vi "RUSHArmControl.vi"(1 "In Cluster":T2) -> (0 "Out Cluster":T1)   [LabVIEW 2012]
panel:
  in  "Setpoint P Gain":dbl=2.0
  in  "Manual P Gain":dbl=2.0
  in  "Vision P Gain":dbl=0.75
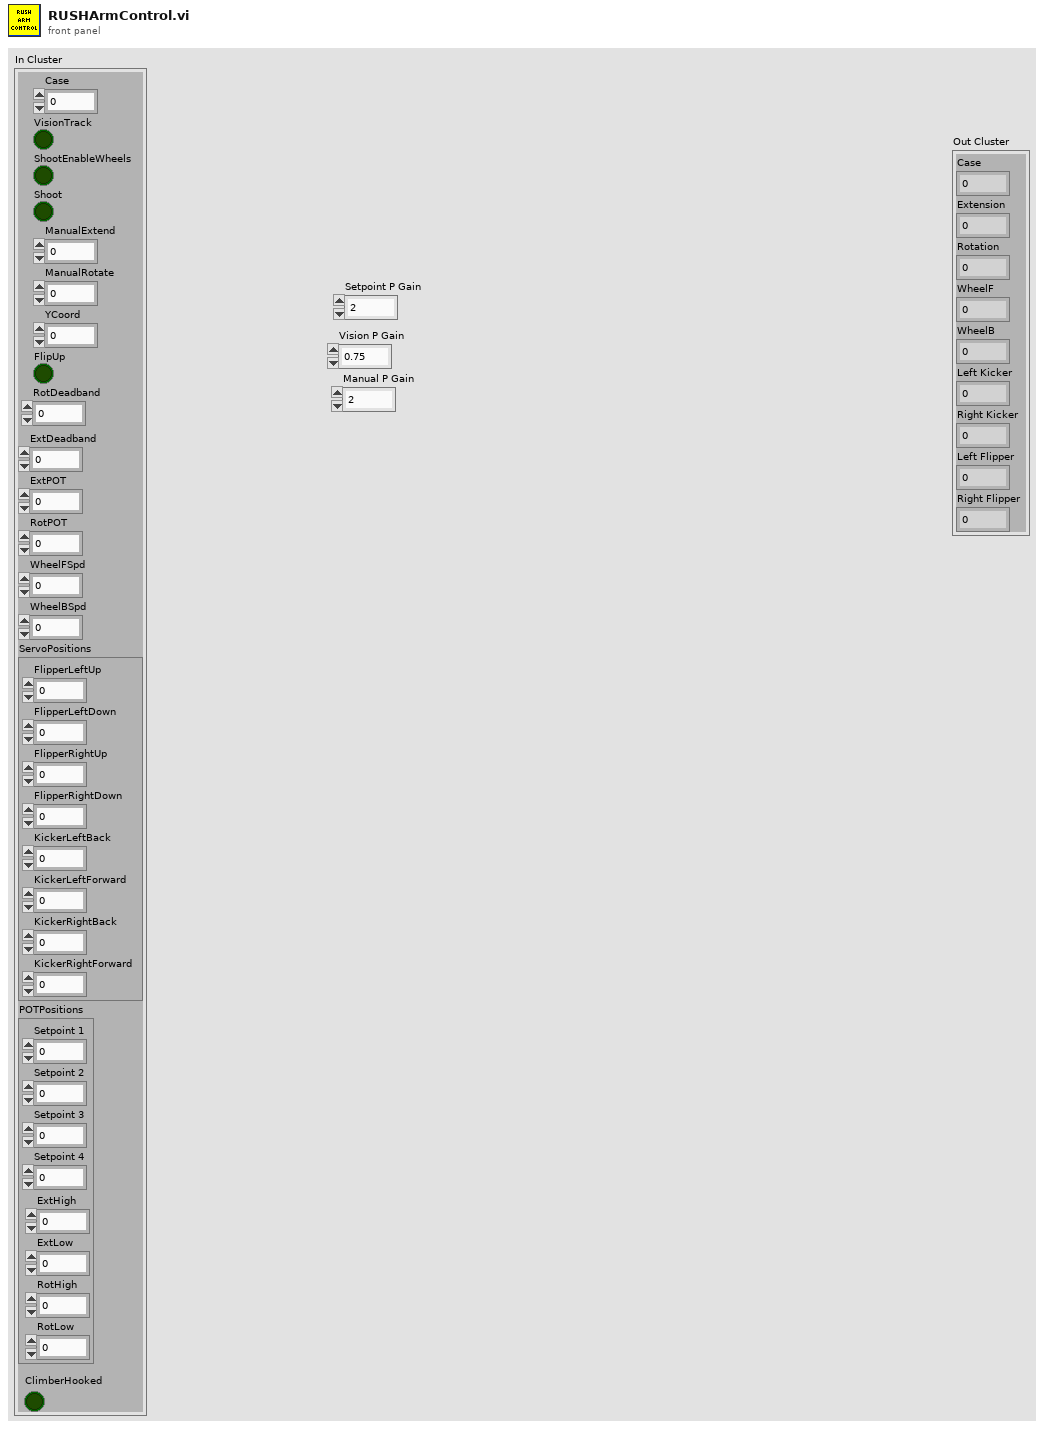
[diagram p1: front panel]
types:
  T1 = cluster{"Case":dbl, "Extension":dbl, "Rotation":dbl, "WheelF":dbl, "WheelB":dbl, "Left Kicker":dbl, "Right Kicker":dbl, "Left Flipper":dbl, "Right Flipper":dbl}
  T2 = cluster{"Case":dbl, "VisionTrack":bool, "ShootEnableWheels":bool, "Shoot":bool, "ManualExtend":dbl, "ManualRotate":dbl, "YCoord":dbl, "FlipUp":bool, "RotDeadband":dbl, "ExtDeadband":dbl, "ExtPOT":dbl, "RotPOT":dbl, "WheelFSpd":dbl, "WheelBSpd":dbl, "ServoPositions":cluster{"FlipperLeftUp":dbl, "FlipperLeftDown":dbl, "FlipperRightUp":dbl, "FlipperRightDown":dbl, "KickerLeftBack":dbl, "KickerLeftForward":dbl, "KickerRightBack":dbl, "KickerRightForward":dbl}, "POTPositions":cluster{"Setpoint 1":dbl, "Setpoint 2":dbl, "Setpoint 3":dbl, "Setpoint 4":dbl, "RotLow":dbl, "RotHigh":dbl, "ExtLow":dbl, "ExtHigh":dbl}, "ClimberHooked":bool}
  T3 = cluster{"FlipperLeftUp":dbl, "FlipperLeftDown":dbl, "FlipperRightUp":dbl, "FlipperRightDown":dbl, "KickerLeftBack":dbl, "KickerLeftForward":dbl, "KickerRightBack":dbl, "KickerRightForward":dbl}
  T4 = cluster{"Setpoint 1":dbl, "Setpoint 2":dbl, "Setpoint 3":dbl, "Setpoint 4":dbl, "RotLow":dbl, "RotHigh":dbl, "ExtLow":dbl, "ExtHigh":dbl}
  T5 = cluster{"t":dbl, "y":dbl, "y":dbl, "Output":dbl, "Output":dbl, "KickerLeftBack":dbl, "KickerRightBack":dbl, "FlipperLeftDown":dbl, "FlipperRightDown":dbl}
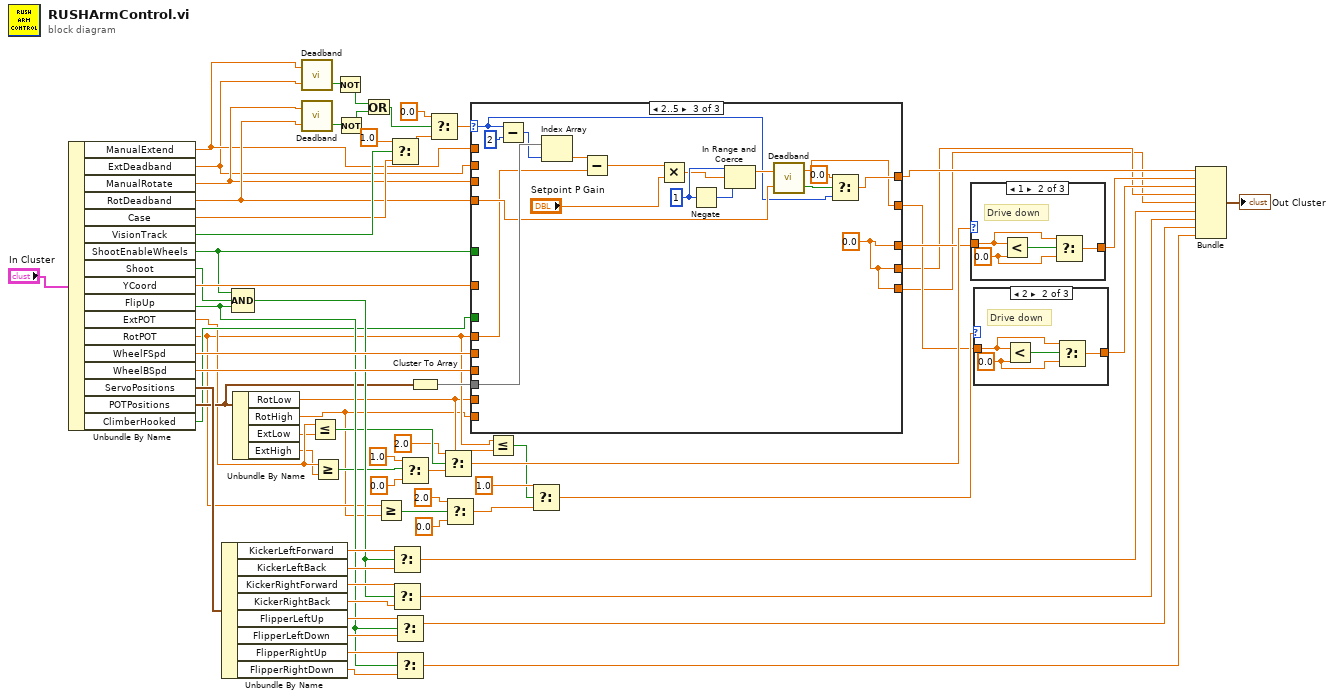
[diagram p0: block diagram]
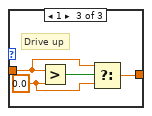
[diagram p3: hidden frame]
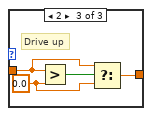
[diagram p5: hidden frame]
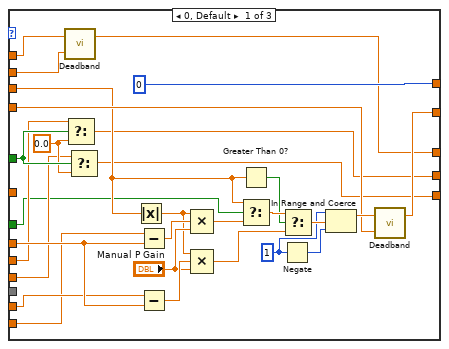
[diagram p6: hidden frame]
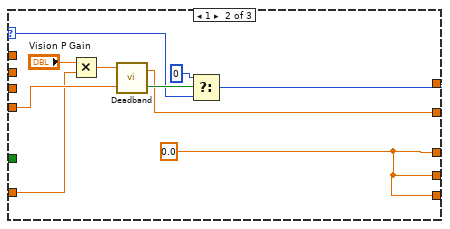
[diagram p7: hidden frame]
diagram:
  n1 = Unbundle By Name("In Cluster") -> ("ManualExtend"=w52:dbl, "ExtDeadband"=w51:dbl, "ManualRotate"=w53:dbl, "RotDeadband"=w55:dbl, "Case"=w56:dbl, "VisionTrack"=w57:bool, "ShootEnableWheels"=w46:bool, "Shoot"=w47:bool, "YCoord"=w54:dbl, "FlipUp"=w36:bool, "ExtPOT"=w27:dbl, "RotPOT"=w15:dbl, "WheelFSpd"=w50:dbl, "WheelBSpd"=w49:dbl, "ServoPositions"=w48:T3, "POTPositions"=w35:T4, "ClimberHooked"=w33:bool)
  n2 = Unbundle By Name(w48) -> ("KickerLeftForward"=w45:dbl, "KickerLeftBack"=w44:dbl, "KickerRightForward"=w43:dbl, "KickerRightBack"=w42:dbl, "FlipperLeftUp"=w40:dbl, "FlipperLeftDown"=w38:dbl, "FlipperRightUp"=w39:dbl, "FlipperRightDown"=w37:dbl)
  n3 = Compound Arithmetic op=AND(w46, w47, w36) -> (w41:bool)
  n4 = Unbundle By Name(w35) -> ("RotLow"=w14:dbl, "RotHigh"=w13:dbl, "ExtLow"=w26:dbl, "ExtHigh"=w25:dbl)
  n5 = call "Deadband.vi"("Deadband"=w51, "Input"=w52) -> ("In Deadband"=w62:bool)  [unwired: 1 out]
  n6 = call "Deadband.vi"("Deadband"=w55, "Input"=w53) -> ("In Deadband"=w61:bool)  [unwired: 1 out]
  n7 = Less Or Equal?(x=w27, y=w26) -> (x <= y?=w28:bool)
  n8 = Greater Or Equal?(x=w27, y=w25) -> (x >= y?=w32:bool)
  n9 = Not(x=w62) -> (.not. x?=w59:bool)
  n10 = Not(x=w61) -> (.not. x?=w60:bool)
  n11 = Or(x=w59, y=w60) -> (x .or. y?=w58:bool)
  n12 = Greater Or Equal?(x=w15, y=w13) -> (x >= y?=w16:bool)
  n13 = Select(t=1.0, s=w57, f=w56) -> (s? t:f=w64:dbl)
  n14 = Select(t=w45, s=w41, f=w44) -> (s? t:f=w5:dbl)
  n15 = Select(t=w43, s=w41, f=w42) -> (s? t:f=w4:dbl)
  n16 = Select(t=w40, s=w36, f=w38) -> (s? t:f=w3:dbl)
  n17 = Select(t=w39, s=w36, f=w37) -> (s? t:f=w2:dbl)
  n18 = Select(t=1.0, s=w32, f=0.0) -> (s? t:f=w29:dbl)
  n19 = Cluster To Array(cluster=w35) -> (array=w34:dbl[])
  n20 = Select(t=0.0, s=w58, f=w64) -> (s? t:f=w67:dbl)
  n21 = Select(t=2.0, s=w28, f=w29) -> (s? t:f=w23:dbl)
  n22 = Select(t=2.0, s=w16, f=0.0) -> (s? t:f=w19:dbl)
  n23 = case shown="2..5" w67 {
    selector: w67 -> [_ w101 w110]
    tunnel: w55 -> [w81 w104 w114]
    tunnel: w54 -> [_ w103 _]
    tunnel: [0 ("t") w99 w109] -> w10
    tunnel: [w79 w98 w108] -> w11
    tunnel: w15 -> [w84 _ w113]
    tunnel: w14 -> [w83 _ _]
    tunnel: w13 -> [w82 _ _]
    tunnel: w53 -> [w80 _ _]
    tunnel: w52 -> [w77 _ _]
    tunnel: w51 -> [w76 _ _]
    tunnel: [w75 w97 w107] -> w22
    tunnel: w46 -> [w74 _ _]
    tunnel: w50 -> [w72 _ _]
    tunnel: w49 -> [w71 _ _]
    tunnel: [w70 w97 w107] -> w7
    tunnel: [w69 w97 w107] -> w6
    tunnel: w34 -> [_ _ w123]
    tunnel: w33 -> [w68 _ _]
    frame 0, Default {
      w73 = 0.0 ("f")
      w86 = 1
      n24 = call "Deadband.vi"("Deadband"=w76, "Input"=w77) -> ("Output"=w75:dbl)  [unwired: 1 out]
      n25 = Select(t=w72, s=w74, f=w73) -> (s? t:f=w70:dbl)
      n26 = Select(t=w71, s=w74, f=w73) -> (s? t:f=w69:dbl)
      n27 = Absolute Value(x=w80) -> (abs(x)=w90:dbl)
      n28 = Subtract(x=w82, y=w84) -> (x-y=w96:dbl)
      n29 = Subtract(x=w83, y=w84) -> (x-y=w95:dbl)
      n30 = Compound Arithmetic op=MULTIPLY(w90, w96, "Manual P Gain") -> (w93:dbl)
      n31 = Compound Arithmetic op=MULTIPLY(w90, w95, "Manual P Gain") -> (w91:dbl)
      n32 = Greater Than 0?(x=w80) -> (x > 0?=w89:bool)
      n33 = Select(t=w80, s=w68, f=w93) -> (s? t:f=w92:dbl)
      n34 = Negate(x=w86) -> (-x=w87:i32)
      n35 = Select(t=w92, s=w89, f=w91) -> (s? t:f=w88:dbl)
      n36 = In Range and Coerce(upper limit=w86, x=w88, lower limit=w87) -> (coerced(x)=w85:dbl)  [unwired: 1 out]
      n37 = call "Deadband.vi"("Deadband"=w81, "Input"=w85) -> ("Output"=w79:dbl)  [unwired: 1 out]
    }
    frame 1 {
      w97 = 0.0 ("Output")
      n38 = Multiply(x="Vision P Gain", y=w103) -> (x*y=w105:dbl)
      n39 = call "Deadband.vi"("Deadband"=w104, "Input"=w105) -> ("In Deadband"=w102:bool, "Output"=w98:dbl)
      n40 = Select(t=0, s=w102, f=w101) -> (s? t:f=w99:i32)
    }
    frame 2..5 {
      w107 = 0.0 ("Output")
      w117 = 1
      n41 = Subtract(x=w110, y=2) -> (x-y=w122:i32)
      n42 = Index Array(array=w123, index=w122) -> (element=w121:dbl)
      n43 = Subtract(x=w121, y=w113) -> (x-y=w120:dbl)
      n44 = Multiply(x=w120, y="Setpoint P Gain") -> (x*y=w116:dbl)
      n45 = Negate(x=w117) -> (-x=w118:i32)
      n46 = In Range and Coerce(upper limit=w117, x=w116, lower limit=w118) -> (coerced(x)=w115:dbl)  [unwired: 1 out]
      n47 = call "Deadband.vi"("Deadband"=w114, "Input"=w115) -> ("In Deadband"=w112:bool, "Output"=w108:dbl)
      n48 = Select(t=0.0, s=w112, f=w110) -> (s? t:f=w109:dbl)
    }
  }
  n49 = Less Or Equal?(x=w15, y=w14) -> (x <= y?=w20:bool)
  n50 = Select(t=1.0, s=w20, f=w19) -> (s? t:f=w12:dbl)
  n51 = case shown="1" w23 {
    tunnel: w22 -> [w125 w127 w131]
    tunnel: [w125 w126 w130] -> w9
    frame 0, Default {
      # "All good"
    }
    frame 1 {
      w128 = 0.0 ("y")
      # "Drive down"
      n52 = Less?(x=w127, y=w128) -> (x < y?=w129:bool)
      n53 = Select(t=w127, s=w129, f=w128) -> (s? t:f=w126:dbl)
    }
    frame 2 {
      w132 = 0.0 ("y")
      # "Drive up"
      n54 = Greater?(x=w131, y=w132) -> (0:w133:bool)
      n55 = Select(t=w131, s=w133, f=w132) -> (s? t:f=w130:dbl)
    }
  }
  n56 = case shown="2" w12 {
    tunnel: w11 -> [w134 w136 w140]
    tunnel: [w134 w135 w139] -> w8
    frame 0, Default {
      # "All good"
    }
    frame 2 {
      w137 = 0.0 ("y")
      # "Drive down"
      n57 = Less?(x=w136, y=w137) -> (x < y?=w138:bool)
      n58 = Select(t=w136, s=w138, f=w137) -> (s? t:f=w135:dbl)
    }
    frame 1 {
      w141 = 0.0 ("y")
      # "Drive up"
      n59 = Greater?(x=w140, y=w141) -> (0:w142:bool)
      n60 = Select(t=w140, s=w142, f=w141) -> (s? t:f=w139:dbl)
    }
  }
  n61 = Bundle("t"=w10, "y"=w9, "y"=w8, "Output"=w7, "Output"=w6, "KickerLeftBack"=w5, "KickerRightBack"=w4, "FlipperLeftDown"=w3, "FlipperRightDown"=w2) -> (→"Out Cluster":T5)  [unwired: 1 in]
